vi "ReplaceError.vi"(5 "ErrorToClear":errorcluster, 9 "SourceError":errorcluster) -> (19 "error out":errorcluster)   [LabVIEW 2020, in "G#IDE.lvlib" / "SupportLib.lvlib"]
uses:
  <resource>/Framework/Providers/AddQ/G#IDE/support/G#IDELib/SupportLib.lvlib
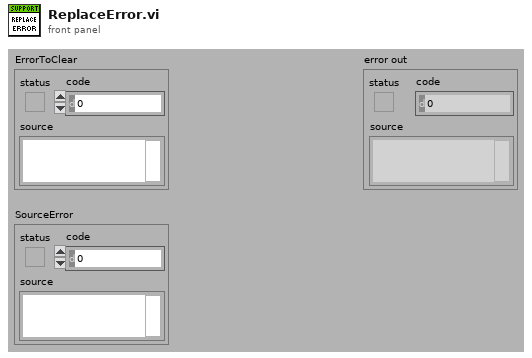
[diagram p1: front panel]
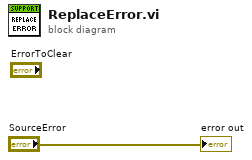
[diagram p0: block diagram]
diagram:
  "error out" <- "SourceError"
